vi "Set Config.vi"(8 "Error In":errorcluster, 11 "object in":refnum<class "PXI-5441.lvclass">) -> (0 "Error Out":errorcluster, 3 "object out":refnum<class "PXI-5441.lvclass">)   [LabVIEW 2023, in "PXI-5441.lvlib" / "PXI-5441.lvclass"]
uses:
  PXI-5441.lvclass
  PXI-5441.lvclass/PXI-5441.ctl
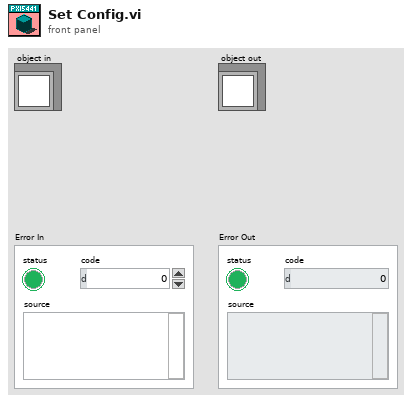
[diagram p1: front panel]
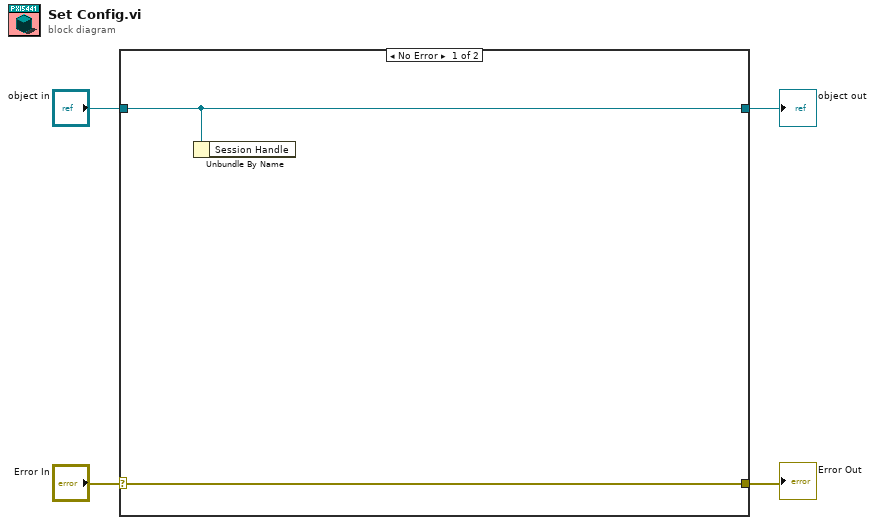
[diagram p0: block diagram]
diagram:
  n1 = case shown="No Error" "Error In" {
    selector: "Error In" -> [w6 w8]
    tunnel: [w6 w8] -> w3
    tunnel: [w5 w7] -> w1
    tunnel: "object in" -> [w5 w7]
    frame No Error {
      n2 = Unbundle By Name(w5) -> ()  [unwired: 1 out]
    }
    frame Error {
    }
  }
  "Error Out" <- w3
  "object out" <- w1
